vi "Process.vi"(8 "error in":errorcluster, 11 "Inst UI.RP100":refnum<class "Inst UI.RP100.lvclass">) -> (0 "error out":errorcluster, 3 "Inst UI.RP100 out":refnum<class "Inst UI.RP100.lvclass">)   [LabVIEW 2019, in "Inst UI.RP100.lvclass"]
doc: "---------------------------------------------------------------\nJKI State Machine Objects™\nhttp://jki.net/state-machine-objects/\nCopyright (C) 2005-2015, JKI <info@jki.net>\nALL RIGHTS RESERVEDJKI State Machine Objects (SMO) 1.0.0.5\nJKI - JKI\nCopyright (c) 2016, JKI"
uses:
  Inst UI.RP100.lvclass
  <vilib>/JKI/JKI SMO/SMO/SMO.lvclass
  <vilib>/JKI/JKI SMO/SMO.UI/SMO.UI.lvclass
  <userlib>/LevyLab/Instrument Framework/SMOs/Instrument/Instrument.lvclass
  Inst.RP100/Typedefs/Inst.RP100.getAll--Cluster.ctl
  Inst.RP100/Inst.RP100.lvclass
  <userlib>/LevyLab/Instrument Framework/SMOs/Instrument UI/Instrument UI.lvclass
  Inst UI.RP100.UI--Cluster.ctl
  <userlib>/LevyLab/Instrument Framework/SMOs/Configuration/Configuration.lvclass
  Inst.RP100/Typedefs/Inst.RP100.Configuration--Cluster.ctl
  <userlib>/LevyLab/Instrument Framework/SMOs/Instrument/Typedefs/Client Type--Enum.ctl
  <userlib>/LevyLab/Instrument Framework/SMOs/RemoteControl/Typedefs/Message--Cluster.ctl
  <userlib>/LevyLab/Instrument Framework/SMOs/RemoteControl/RemoteControl.lvclass
  09e9697b-516c-49fb-b2dc-692589121b6f.vi
  C:/Program Files (x86)/National Instruments/LabVIEW 2019/user.lib/LevyLab/Instrument Framework/SMOs/Instrument UI/Instrument UI.lvclass
  C:/Program Files (x86)/National Instruments/LabVIEW 2019/vi.lib/JKI/JKI SMO/SMO.UI/SMO.UI.lvclass
  C:/Program Files (x86)/National Instruments/LabVIEW 2019/vi.lib/JKI/JKI SMO/SMO/SMO.lvclass
  C:/Program Files (x86)/National Instruments/LabVIEW 2019/user.lib/LevyLab/Instrument Framework/Instrument Types/VSource/Instrument.VSource.lvclass
  C:/Program Files (x86)/National Instruments/LabVIEW 2019/user.lib/LevyLab/Instrument Framework/SMOs/Instrument/Instrument.lvclass
  Inst.RP100/Typedefs/Output State--Enum.ctl
  RP100/RP100.lvclass
  Inst.RP100/Typedefs/Output Channel--Enum.ctl
panel:
  in  "Go to Setpoint":bool
  in  "Enable Output":bool
  in  "Slew (V/s)":dbl=0.0001 min=0.0001 max=100.0 format="%#_6p"
  in  "Ch2 (V)":dbl min=-200.0 max=200.0
  in  "Ch1 (V)":dbl min=-200.0 max=200.0
  out "Bridge Titles":string="C\nC =\nLoss=\nV ="
  out "Bridge Status":string="Bridge:NaNpF\n0.000000nS\n0.000000V"
  out "Ch 2 status":string="Channel 2:Shorted\n0.0V\n0.0V\n0.0V\n0.0A"
  out "Ch 1 Status":string="Channel 1:Shorted\n0.0V\n0.0V\n0.0V\n0.0A"
  out "RP100 Titles":string="RP100\nState =\nLevel =\nSlew =\nMeasured V =\nMeasured I ="
  out "Status":string="SMO State: Stopped"
  out "version":string="vDevelopment"
  # "Razorbill Monitor & Control"
  # "Actions"
  # "Setpoints"
  # "RP100 Status"
  # "Bridge Status"
  # "SMO UI Template"
  # "For instructions on how to use the JKI State Machine Objects, examples and video tutorials, visit:\nhttp://jki.net/state-machine-objects/\n\nJKI State Machine Objects™\nhttp://jki.net/state-machine-objects/\nCopyright (C) 2005-2015, JKI <info@jki.net>\nALL RIGHTS RESERVED"
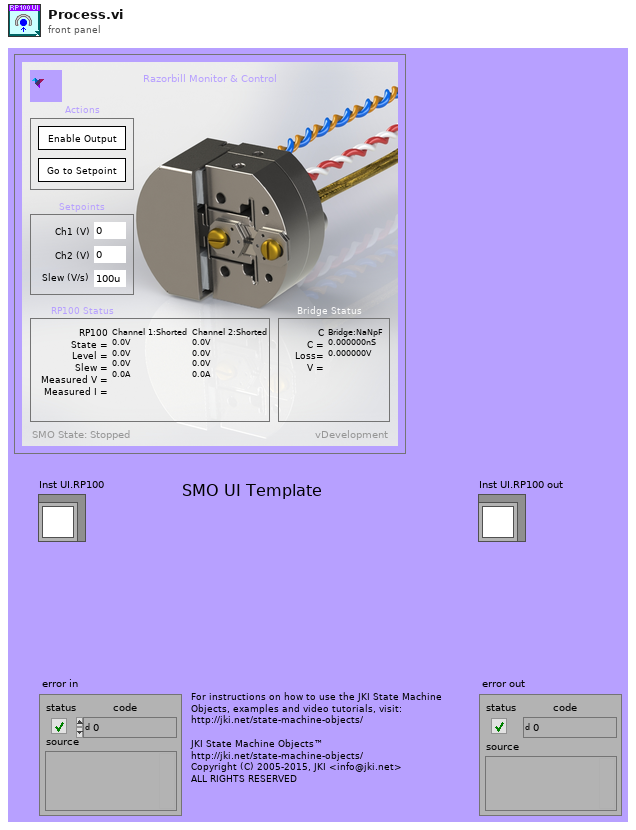
[diagram p1: front panel]
types:
  T1 = typedef "Inst.RP100.lvclass/Output State--Enum.ctl" = enum16{"Shorted", "Enabled"}
  T2 = typedef "Inst.RP100.lvclass/Output Channel--Enum.ctl" = enum16{"Output 1", "Output 2"}
  T3 = enum32{"invalid app kind", "Development System", "Run Time System", "Student Edition", "Embedded LabVIEW", "Evaluation", "Custom"}
  T4 = enum32{"Invalid", "Standard", "Closed", "Hidden", "Minimized", "Maximized"}
  T5 = typedef "Instrument.lvclass/Client Type--Enum.ctl" = enum16{"Remote", "Local"}
  T6 = typedef "RemoteControl.lvclass/Message--Cluster.ctl" = cluster{"Command":string, "Data":variant, "ID":string}
  T7 = typedef "Inst.RP100.lvclass/Inst.RP100.Configuration--Cluster.ctl" = cluster{"Example Setting 1":dbl, "Example Setting 2":dbl, "Example Setting 3":string}
  T8 = typedef "Inst.RP100.lvclass/Inst.RP100.getAll--Cluster.ctl" = cluster{"Output State Ch1":string, "Output State Ch2":string, "Level (V) Ch1":dbl, "Level (V) Ch2":dbl, "Slew (V/s) Ch1":dbl, "Slew (V/s) Ch2":dbl, "measured V (V) Ch1":dbl, "measured V (V) Ch2":dbl, "measured I (A) Ch1":dbl, "measured I (A) Ch2":dbl}
  T9 = typedef "Inst UI.RP100.lvclass/Inst UI.RP100.UI--Cluster.ctl" = cluster{"Ch1 (V)":dbl, "Ch2 (V)":dbl, "Slew (V/s)":dbl}
  T10 = cluster{"Core":cluster{"Current VI Reference":refnum<vi>, "Close Panel on Exit?":bool, "Last Error":cluster{"error":errorcluster, "previous state":string, "remaining states":string}, "Shutdown?":bool}, "Instrument UI":refnum<class "Inst UI.RP100.lvclass">, "Instrument":refnum<class "Inst.RP100.lvclass">, "Configuration":refnum<class "Configuration.lvclass">, "Config Cluster":T7, "getAll":T8, "UI Cluster":T9, "Message":T6}
  T11 = typedef "SMO.lvclass/SMOState --Enum.ctl" = enum16{"unknown", "Created", "Started", "Stopped"}
  T12 = cluster{"Current VI Reference":refnum<vi>, "Close Panel on Exit?":bool, "Last Error":cluster{"error":errorcluster, "previous state":string, "remaining states":string}, "Shutdown?":bool}
  T13 = typedef "SMO.lvclass/Protected Events.ctl" = cluster{"StopProcesses":refnum<user-event>, "AbortProcesses":refnum<user-event>, "Config Changed":refnum<user-event>, "Dependency":refnum<user-event>}
  T14 = typedef "Instrument.lvclass/PublicEvents--Cluster.ctl" = cluster{"MessageFromProcess":refnum<user-event>}
  T15 = typedef "Inst.RP100.lvclass/PublicEvents--Cluster.ctl" = cluster{"MessageFromProcess":refnum<user-event>}
  T16 = typedef "SMO.lvclass/Public Events.ctl" = cluster{"Error":refnum<user-event>, "State":refnum<user-event>, "Reserve State":refnum<user-event>}
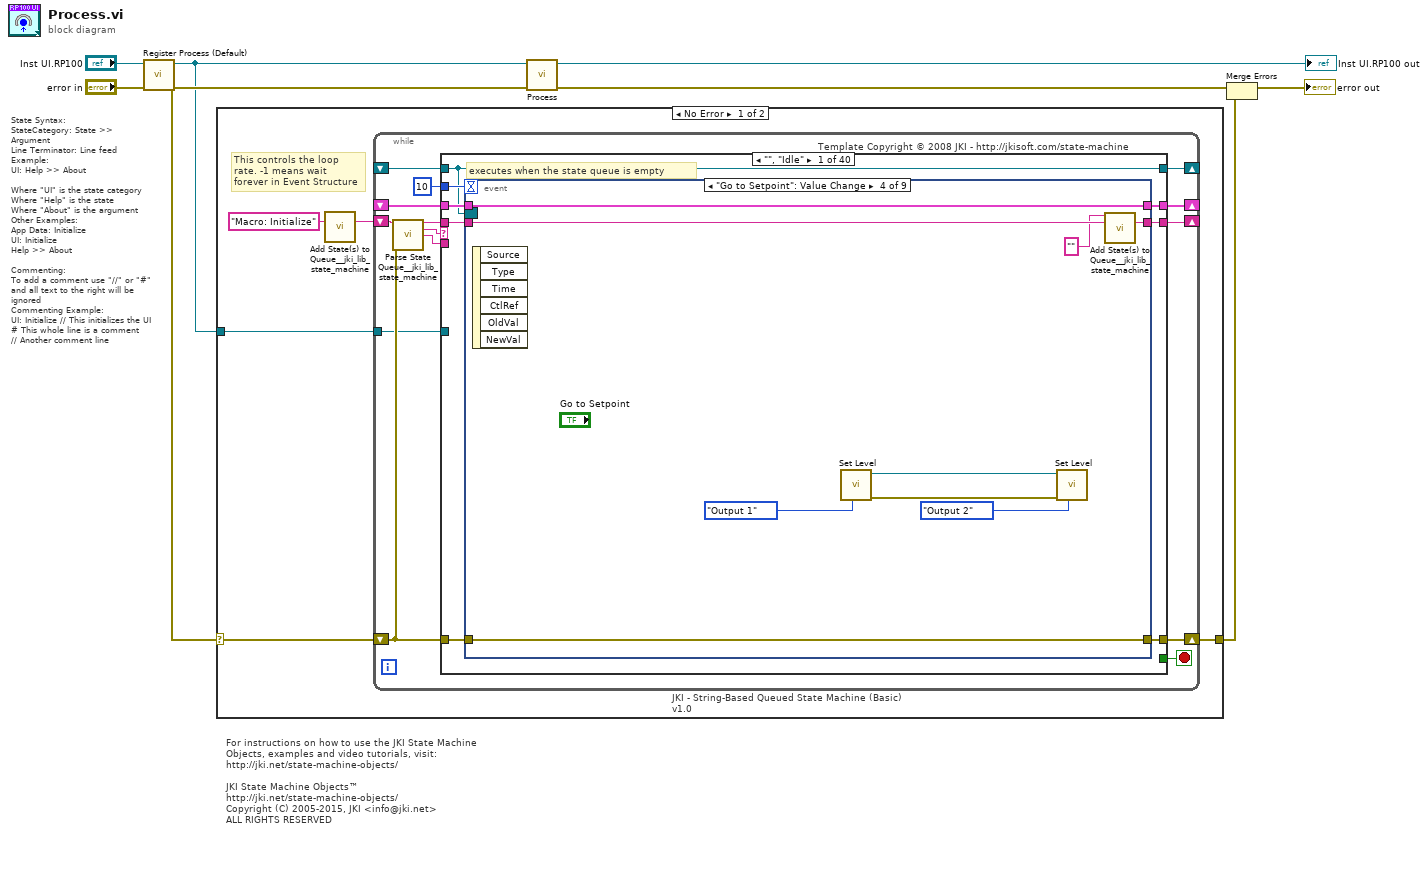
[diagram p0: block diagram]
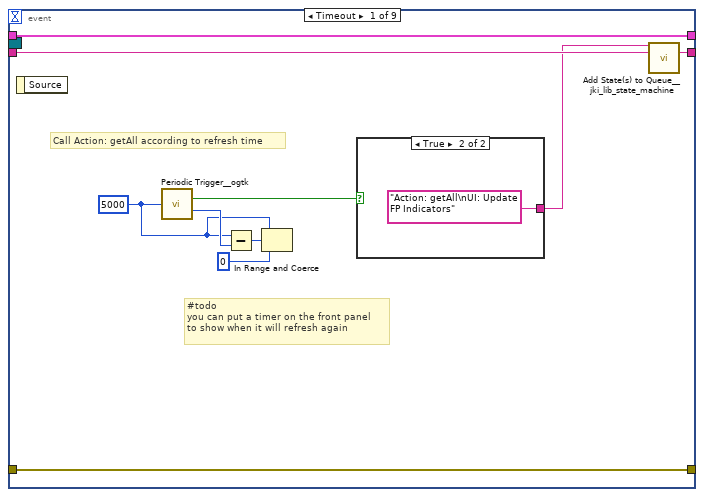
[diagram p2: hidden frame]
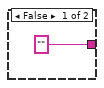
[diagram p3: hidden frame]
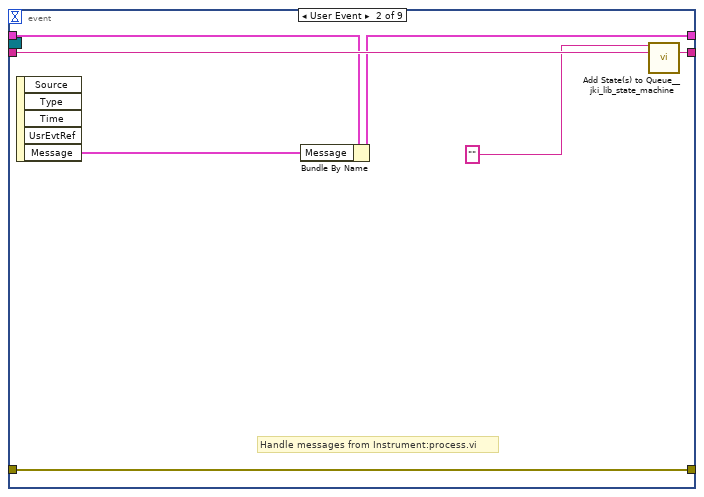
[diagram p4: hidden frame]
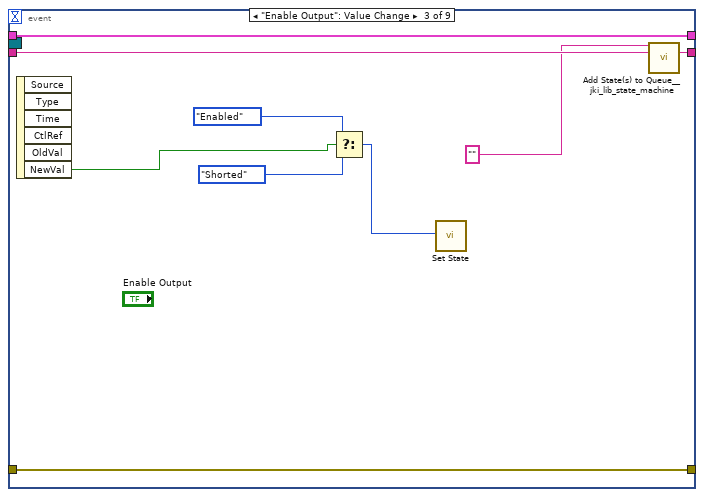
[diagram p5: hidden frame]
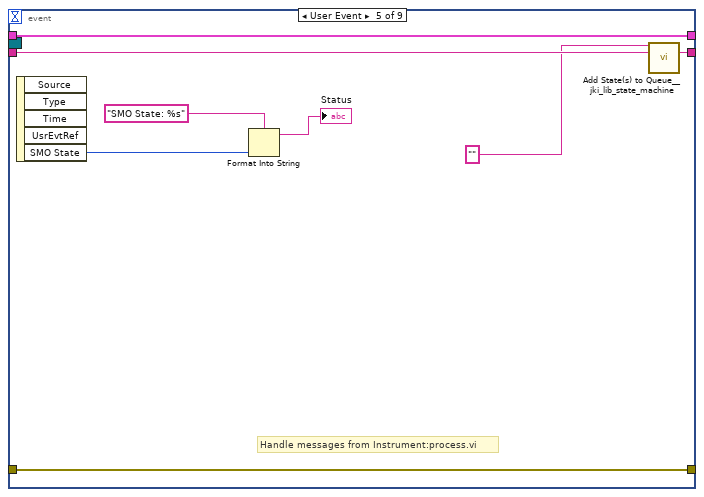
[diagram p6: hidden frame]
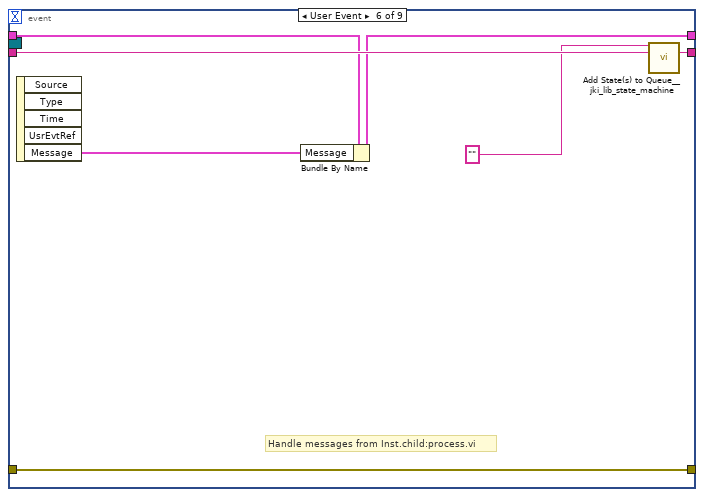
[diagram p7: hidden frame]
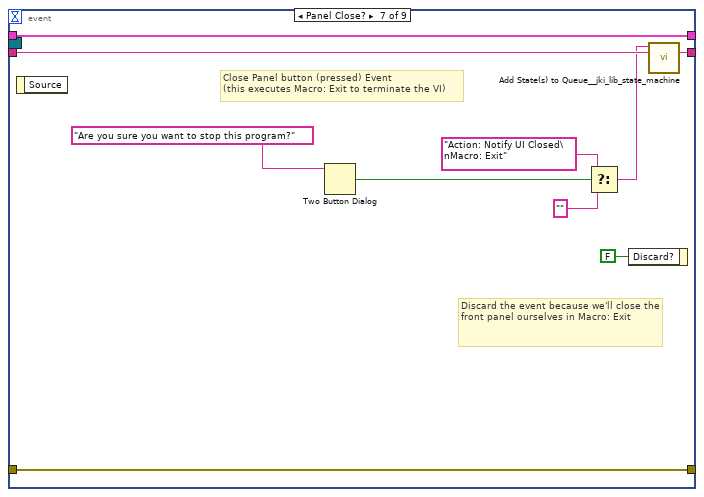
[diagram p8: hidden frame]
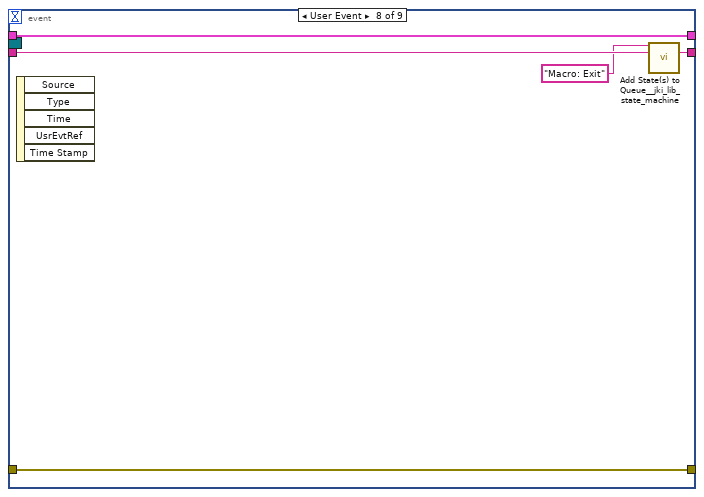
[diagram p9: hidden frame]
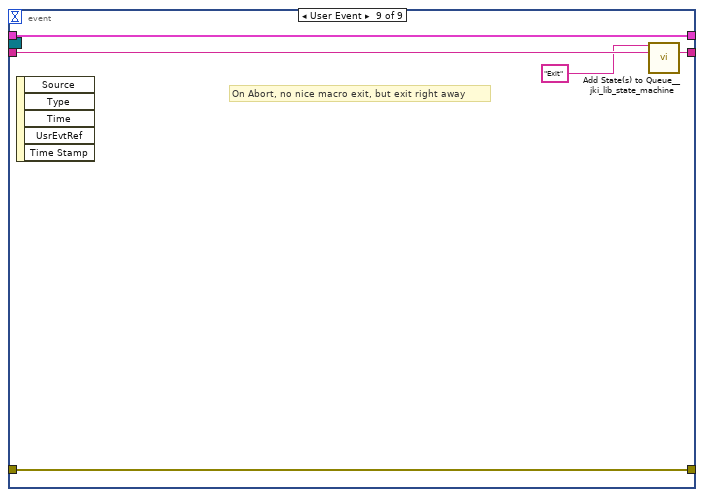
[diagram p10: hidden frame]
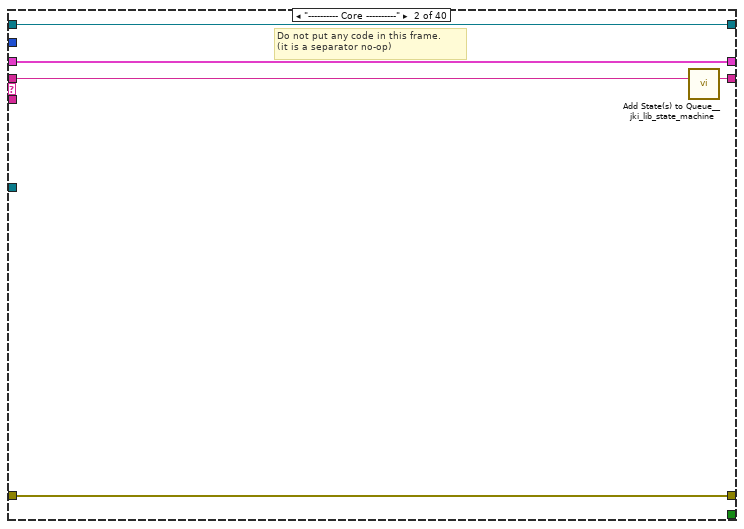
[diagram p11: hidden frame]
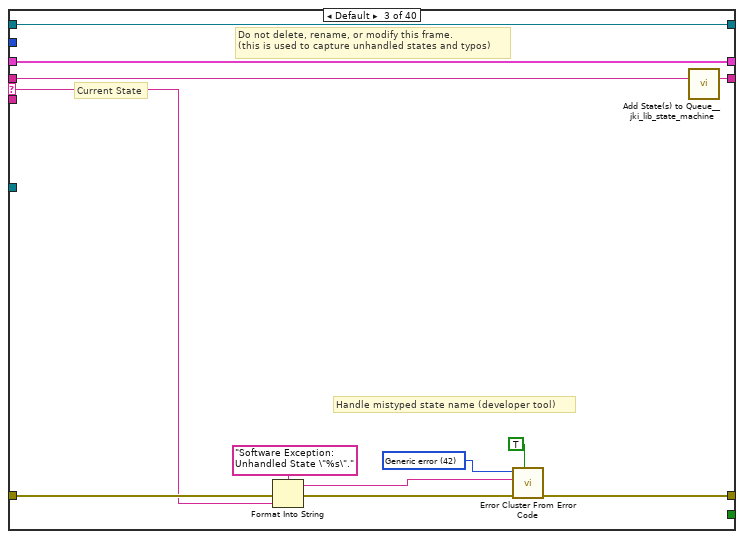
[diagram p12: hidden frame]
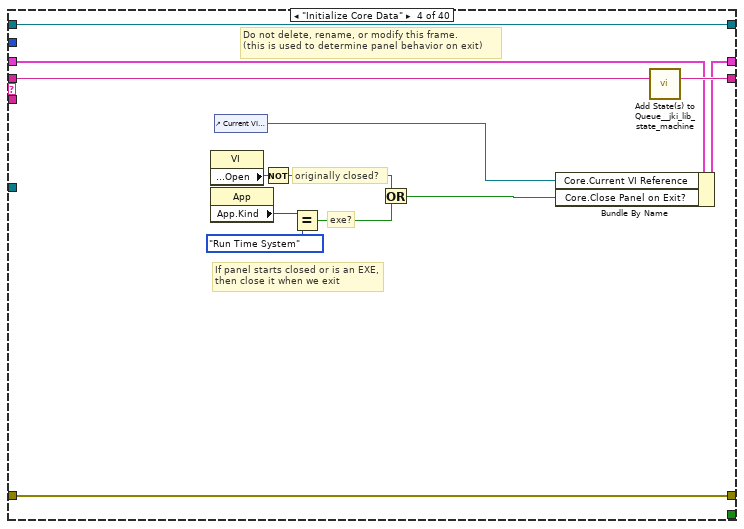
[diagram p13: hidden frame]
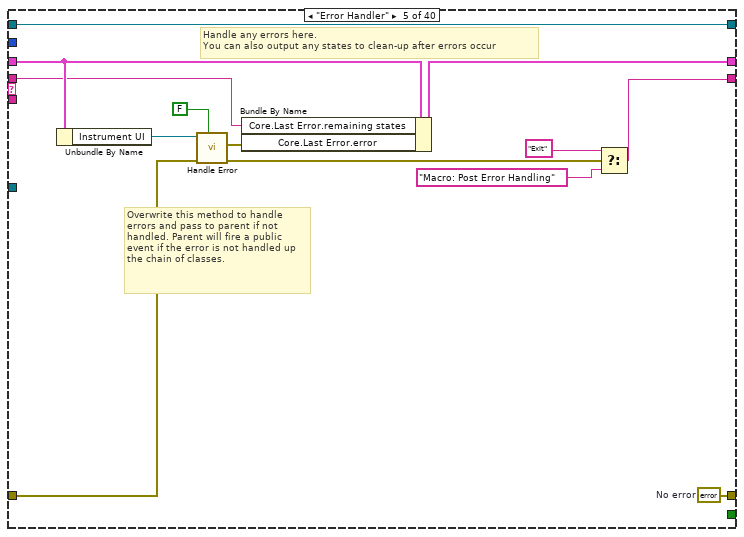
[diagram p14: hidden frame]
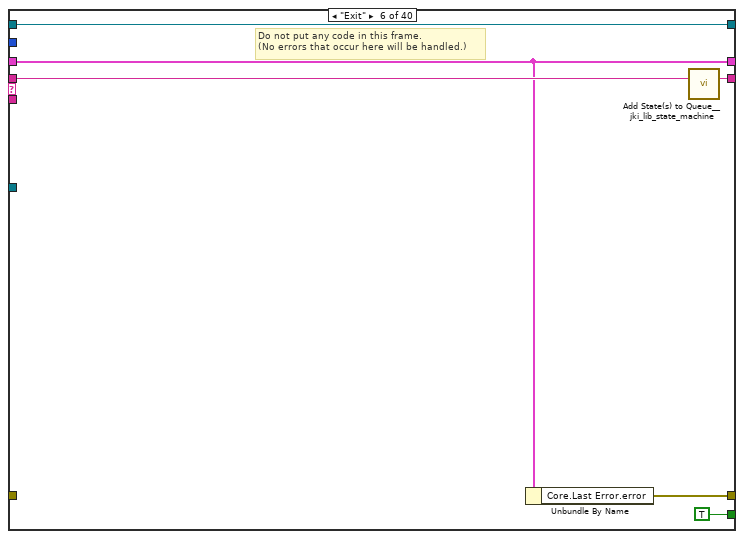
[diagram p15: hidden frame]
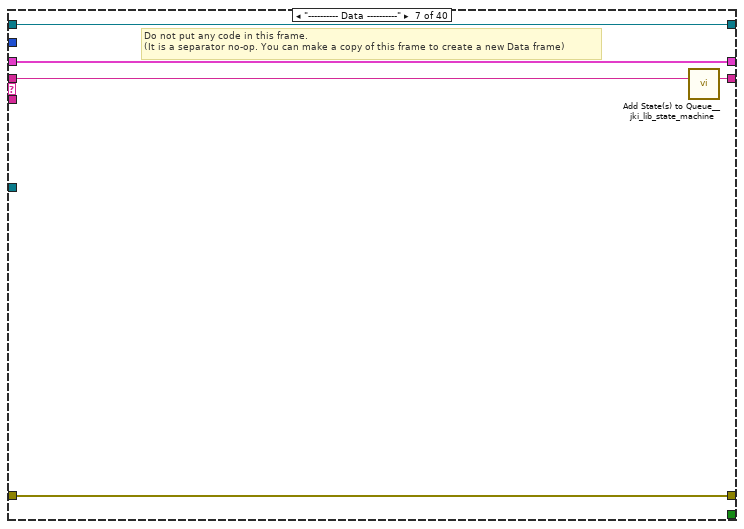
[diagram p16: hidden frame]
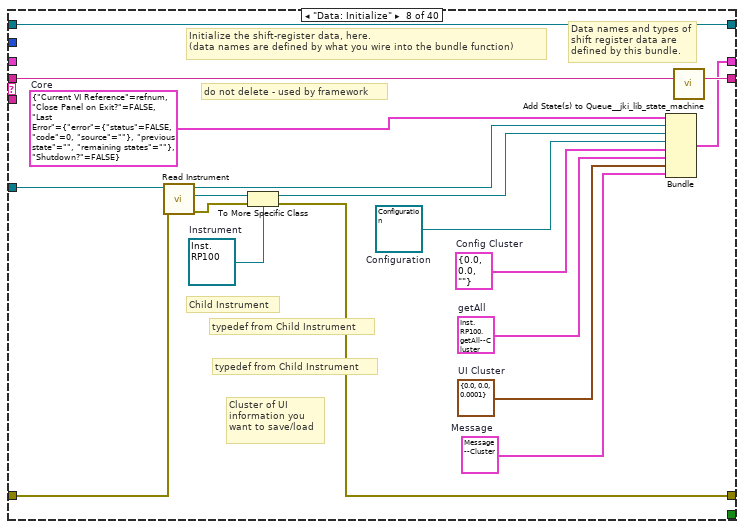
[diagram p17: hidden frame]
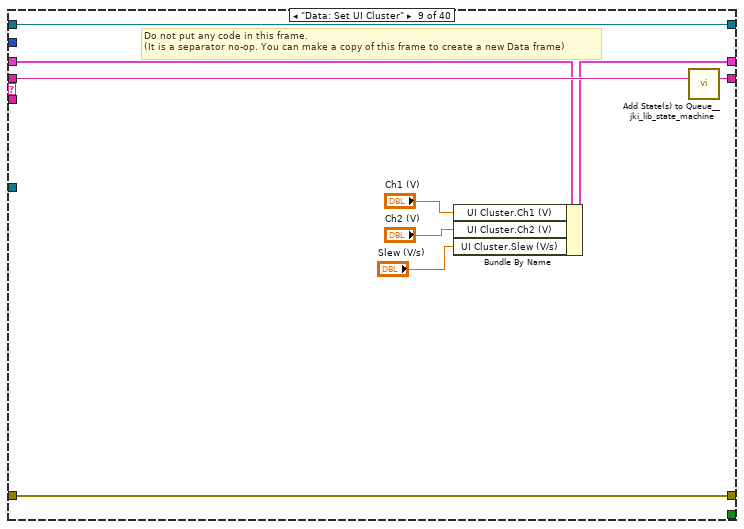
[diagram p18: hidden frame]
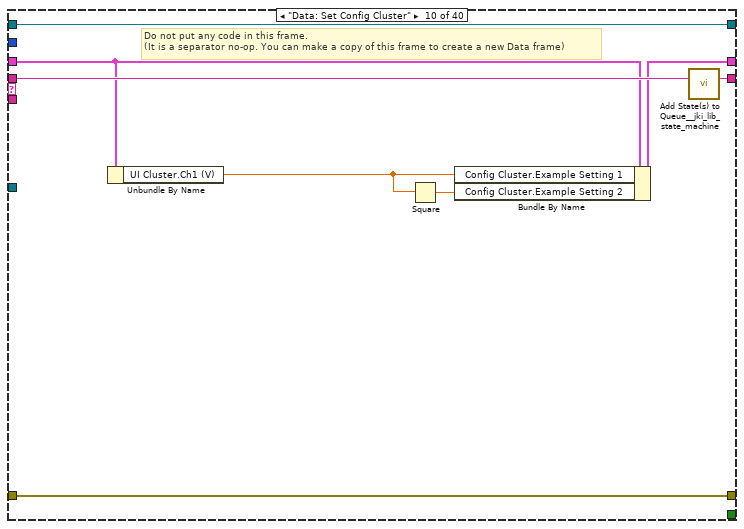
[diagram p19: hidden frame]
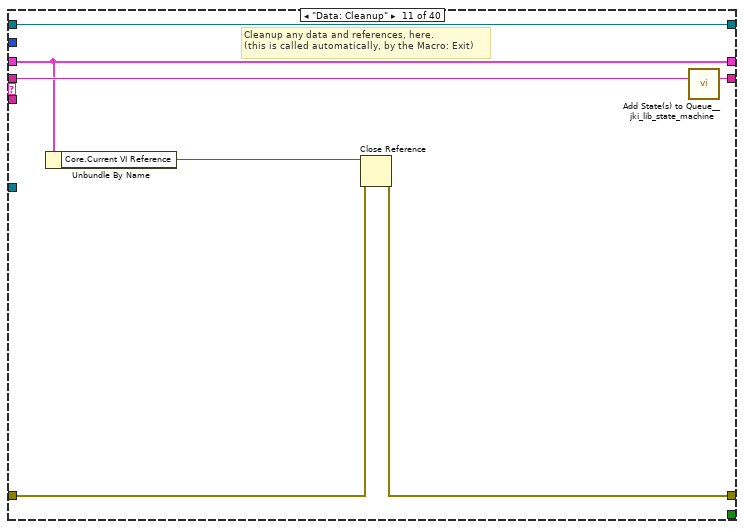
[diagram p20: hidden frame]
diagram:
  # "State Syntax:\nStateCategory: State >> Argument\nLine Terminator: Line feed\nExample:\nUI: Help >> About\n\nWhere \"UI\" is the state category\nWhere \"Help\" is the state\nWhere \"About\" is the argument\nOther Examples:\nApp Data: Initialize\nUI: Initialize\nHelp >> About\n\nCommenting:\nTo add a comment use \"//\" or \"#\" and all text to the right will be ignored\nCommenting Example:\nUI: Initialize // This initializes the UI\n# This whole line is a comment\n// Another comment line"
  # "For instructions on how to use the JKI State Machine Objects, examples and video tutorials, visit:\nhttp://jki.net/state-machine-objects/\n\nJKI State Machine Objects™\nhttp://jki.net/state-machine-objects/\nCopyright (C) 2005-2015, JKI <info@jki.net>\nALL RIGHTS RESERVED"
  n1 = call <vilib>:"Register Process (Default).vi"("error in (no error)"="error in", "SMO"="Inst UI.RP100") -> ("error out"=w5:errorcluster, "SelfRef"=w4:refnum<class "Inst UI.RP100.lvclass">)  [unwired: 8 in]
  n2 = case shown="No Error" w5 {
    selector: w5 -> [w10 w525]
    tunnel: w4 -> [w11 _]
    tunnel: [w9 w525] -> w1
    frame No Error {
      # "This controls the loop rate. -1 means wait forever in Event Structure"
      n3 = call <vilib>:"Add State(s) to Queue__jki_lib_state_machine.vi"("State(s) in (\"\")"="Macro: Initialize") -> ("States Out"=w13:string)  [unwired: 14 in]
      n4 = while "JKI - String-Based Queued State Machine (Basic) v1.0" {
        shift-right: [w20] -> _
        shift-left: _ -> [w19]
        shift-right: [w23] -> w9
        shift-left: w10 -> [w17]
        shift-right: [w22] -> _
        shift-left: w13 -> [w24]
        tunnel: w11 -> [w16]
        shift-right: [w15] -> _
        shift-left: _ -> [w14]
        stop <- w21 stop-if-true
        # "Template Copyright © 2008 JKI - http://jkisoft.com/state-machine"
        n5 = call <vilib>:"Parse State Queue__jki_lib_state_machine.vi"("State Queue"=w24, "Error In (no error)"=w17) -> ("Remaining States"=w26:string, "Current State"=w27:string, "Arguments"=w25:string)  [unwired: 11 in]
        n6 = case shown="\"\", \"Idle\"" w27 {
          selector: w27 -> [_ _ w114 _ _ _ _ _ _ _ _ _ _ _ _ _ _ _ _ _ _ _ _ _ _ _ _ _ _ _ _ _ _ _ _ _ _ _ _ _]
          tunnel: w26 -> [w35 w112 w118 w137 w141 w156 w161 w179 w188 w196 w203 w208 w220 w228 w255 w262 w278 w310 w319 w331 w341 w347 w362 w367 w378 w385 w390 w409 w415 w420 w435 w443 w455 w462 w469 w481 w494 w504 w514 w524]
          tunnel: w25 -> [_ _ _ _ _ _ _ _ _ _ _ _ _ _ _ w256 w272 _ _ _ _ _ _ _ _ _ _ _ _ _ _ _ _ _ _ _ _ _ _ _]
          tunnel: w19 -> [w33 w109 w116 w128 w144 w152 w158 _ w184 w192 w197 w205 w218 w224 w251 w260 w274 w307 w315 w321 w338 w344 w349 w364 w375 w380 w387 w407 w413 w417 w428 w440 w446 w457 w463 w473 w488 w496 w509 w519]
          tunnel: [w32 w110 w120 w134 w146 w151 w159 w166 w186 w194 w199 w206 w215 w226 w252 w257 w275 w308 w317 w329 w339 w345 w360 w365 w369 w381 w388 w404 w410 w418 w421 w438 w447 w459 w464 w478 w491 w501 w505 w515] -> w23
          tunnel: w17 -> [w31 w110 w119 w134 w140 _ w159 w163 w186 w194 w200 w206 w216 w226 w252 w258 w276 w308 w317 w329 w339 w345 w360 w365 w370 w382 w388 w394 w411 w418 w430 w436 w448 w459 w465 w474 w483 w497 w506 w516]
          tunnel: [w34 w111 w117 w136 w138 w155 w160 w178 w187 w195 w202 w207 w219 w227 w254 w261 w277 w309 w318 w330 w340 w346 w361 w366 w377 w384 w389 w408 w414 w419 w434 w442 w454 w461 w468 w480 w493 w503 w513 w523] -> w22
          tunnel: [_ _ _ _ _ TRUE _ _ _ _ _ _ _ _ _ _ _ _ _ _ _ _ _ _ _ _ _ _ _ _ _ _ _ _ _ _ _ _ _ _] -> w21
          tunnel: [w30 w109 w116 w135 w143 w152 w158 w177 w183 w191 w197 w205 w218 w224 w251 w260 w274 w307 w315 w322 w338 w344 w349 w364 w375 w380 w387 w407 w413 w417 w432 w440 w444 w456 w463 w475 w489 w498 w510 w520] -> w20
          tunnel: 10 ("Timeout") -> [w29 _ _ _ _ _ _ _ _ _ _ _ _ _ _ _ _ _ _ _ _ _ _ _ _ _ _ _ _ _ _ _ _ _ _ _ _ _ _ _]
          tunnel: w16 -> [_ _ _ _ _ _ _ w164 _ _ _ _ _ _ _ _ _ _ _ _ _ _ _ _ _ _ _ _ _ _ _ _ _ _ _ _ _ _ _ _]
          tunnel: [w28 w108 w113 w125 w150 w153 w157 w176 w185 w193 w198 w204 w217 w225 w253 w259 w271 w306 w316 w328 w337 w343 w354 w363 w376 w383 w386 w406 w412 w416 w433 w441 w453 w460 w467 w479 w492 w502 w512 w522] -> w15
          tunnel: w14 -> [w28 w108 w113 w125 w150 w153 w157 w176 w185 w193 w198 w204 w217 w225 w253 w259 w271 w306 w316 w328 w337 w343 w354 w363 w376 w383 w386 _ w412 w416 w433 w441 w453 w460 w467 w479 w492 w502 w512 w522]
          frame "", "Idle" {
            # "executes when the state queue is empty"
            n7 = event shown="[3] \"Go to Setpoint\": Value Change" {
              selector: w28 -> [_ _ _ _ _ _ _ _ _]
              dyn-events: _ -> [_ _ _ _ _ _ _ _ _]
              timeout: w29 -> [_ _ _ _ _ _ _ _ _]
              tunnel: w35 -> [w45 w54 w63 w72 w80 w87 w97 w102 w107]
              tunnel: [w44 w53 w62 w71 w79 w86 w96 w101 w106] -> w34
              tunnel: w33 -> [w42 w51 w59 w69 w76 w84 w94 w99 w104]
              tunnel: [w43 w52 w61 w70 w78 w85 w93 w100 w105] -> w32
              tunnel: w31 -> [w43 w52 w61 w70 w78 w85 w93 w100 w105]
              tunnel: [w42 w50 w59 w69 w76 w83 w94 w99 w104] -> w30
              event Timeout {
                w37 = u32 5000 ("time (ms)")
                # "#todo\nyou can put a timer on the front panel\nto show when it will refresh again"
                # "Call Action: getAll according to refresh time"
                n8 = event-data() -> ()  [unwired: 1 in, 1 out]
                n9 = call <userlib>:"Periodic Trigger__ogtk.vi"("time (ms)"=w37) -> ("Triggered"=w40:bool, "timer value"=w39:u32)  [unwired: 12 in, 1 out]
                n10 = Subtract(x=w37, y=w39) -> (x-y=w38:u32)
                n11 = In Range and Coerce(upper limit=w37, x=w38, lower limit=u32 0) -> ()  [unwired: 2 out]
                n12 = case shown="True" w40 {
                  tunnel: ["" ("State(s) in Front (\"\")") "Action: getAll\nUI: Update FP Indicators" ("State(s) in Front (\"\")")] -> w41
                  frame False {
                  }
                  frame True {
                  }
                }
                n13 = call <vilib>:"Add State(s) to Queue__jki_lib_state_machine.vi"("State(s) in Front (\"\")"=w41, "State(s) in (\"\")"=w45) -> ("States Out"=w44:string)  [unwired: 13 in]
              }
              event User Event {
                # "Handle messages from Instrument:process.vi"
                n14 = event-data() -> ("Message"=w48:T6)  [unwired: 1 in, 4 out]
                n15 = Bundle By Name(cluster=w51, "Message"=w48) -> (w50:T10)
                n16 = call <vilib>:"Add State(s) to Queue__jki_lib_state_machine.vi"("State(s) in Front (\"\")"="" ("State(s) in Front (\"\")"), "State(s) in (\"\")"=w54) -> ("States Out"=w53:string)  [unwired: 13 in]
              }
              event "Enable Output": Value Change {
                n17 = event-data() -> ("NewVal"=w55:bool)  [unwired: 1 in, 5 out]
                n18 = Select(t=Output_State--Enum."Enabled" ("Output"), s=w55, f=Output_State--Enum."Shorted" ("Output")) -> (s? t:f=w56:T1)
                n19 = call-dynamic "Set State.vi"("Output"=w56) -> ()  [unwired: 9 in, 2 out]
                n20 = call <vilib>:"Add State(s) to Queue__jki_lib_state_machine.vi"("State(s) in Front (\"\")"="" ("State(s) in Front (\"\")"), "State(s) in (\"\")"=w63) -> ("States Out"=w62:string)  [unwired: 13 in]
              }
              event "Go to Setpoint": Value Change {
                n21 = event-data() -> ()  [unwired: 1 in, 6 out]
                n22 = call-dynamic "Set Level.vi"("Output Channel"=Output_Channel--Enum."Output 1") -> ("error out"=w64:errorcluster, "RP100 out"=w67:refnum<class "RP100.lvclass">)  [unwired: 9 in]
                n23 = call-dynamic "Set Level.vi"("Output Channel"=Output_Channel--Enum."Output 2", "error in (no error)"=w64, "RP100 in"=w67) -> ()  [unwired: 7 in, 2 out]
                n24 = call <vilib>:"Add State(s) to Queue__jki_lib_state_machine.vi"("State(s) in Front (\"\")"="" ("State(s) in Front (\"\")"), "State(s) in (\"\")"=w72) -> ("States Out"=w71:string)  [unwired: 13 in]
              }
              event User Event {
                # "Handle messages from Instrument:process.vi"
                n25 = event-data() -> ("SMO State"=w74:T11)  [unwired: 1 in, 4 out]
                n26 = Format Into String(format string="SMO State: %s", w74) -> (resulting string=→"Status":string)  [unwired: 2 in, 1 out]
                n27 = call <vilib>:"Add State(s) to Queue__jki_lib_state_machine.vi"("State(s) in Front (\"\")"="" ("State(s) in Front (\"\")"), "State(s) in (\"\")"=w80) -> ("States Out"=w79:string)  [unwired: 13 in]
              }
              event User Event {
                # "Handle messages from Inst.child:process.vi"
                n28 = event-data() -> ("Message"=w81:T6)  [unwired: 1 in, 4 out]
                n29 = Bundle By Name(cluster=w84, "Message"=w81) -> (w83:T10)
                n30 = call <vilib>:"Add State(s) to Queue__jki_lib_state_machine.vi"("State(s) in Front (\"\")"="" ("State(s) in Front (\"\")"), "State(s) in (\"\")"=w87) -> ("States Out"=w86:string)  [unwired: 13 in]
              }
              event Panel Close? {
                # "Discard the event because we'll close the front panel ourselves in Macro: Exit"
                # "Close Panel button (pressed) Event\n(this executes Macro: Exit to terminate the VI)"
                n31 = event-data() -> ()  [unwired: 1 in, 1 out]
                n32 = Two Button Dialog(message="Are you sure you want to stop this program?") -> (T button?=w92:bool)  [unwired: 2 in]
                n33 = Select(t="Action: Notify UI Closed\nMacro: Exit", s=w92, f="") -> (s? t:f=w89:string)
                n34 = event-data("Discard?"=FALSE) -> ()  [unwired: 1 in, 1 out]
                n35 = call <vilib>:"Add State(s) to Queue__jki_lib_state_machine.vi"("State(s) in Front (\"\")"=w89, "State(s) in (\"\")"=w97) -> ("States Out"=w96:string)  [unwired: 13 in]
              }
              event User Event {
                n36 = event-data() -> ()  [unwired: 1 in, 5 out]
                n37 = call <vilib>:"Add State(s) to Queue__jki_lib_state_machine.vi"("State(s) in Front (\"\")"="Macro: Exit", "State(s) in (\"\")"=w102) -> ("States Out"=w101:string)  [unwired: 13 in]
              }
              event User Event {
                # "On Abort, no nice macro exit, but exit right away"
                n38 = event-data() -> ()  [unwired: 1 in, 5 out]
                n39 = call <vilib>:"Add State(s) to Queue__jki_lib_state_machine.vi"("State(s) in Front (\"\")"="Exit", "State(s) in (\"\")"=w107) -> ("States Out"=w106:string)  [unwired: 13 in]
              }
            }
          }
          frame "---------- Core ----------" {
            # "Do not put any code in this frame.\n(it is a separator no-op)"
            n40 = call <vilib>:"Add State(s) to Queue__jki_lib_state_machine.vi"("State(s) in (\"\")"=w112) -> ("States Out"=w111:string)  [unwired: 14 in]
          }
          frame Default {
            w123 = 42 items=["No error", "Argument error", "Memory is full", "Out of zone", "End of file", "File already open", "Generic file I/O error", "File not found", "File permission error", "Disk is full", "Duplicate path", "Too many files open", "System feature not enabled", "Resource file not found", "Cannot add resource", "Resource not found", "Image not found", "Image memory error", "Pen does not exist", "Config type invalid", "Config token not found", "Config parse error", "Config memory error", "Bad external code format", "Bad external code offset", "External code not present", "Null window", "Destroy window error", "Null menu", "Print aborted", "Bad print record", "Print driver error", "Windows error during printing", "Memory error during printing", "Print dialog error", "Generic print error", "Invalid device refnum", "Device not found", "Device parameter error", "Device unit error", "Cannot open device", "Device call aborted", "Generic error", "Cancelled by user", "Object ID too low", "Object ID too high", "Object not in heap", "Unknown heap", "Unknown object (invalid DefProc)", "Unknown object (DefProc not in table)", "Message out of range", "Invalid (null) method", "Unknown message", "Manager call not supported", "Bad address", "Network operation in progress", "Network operation timed out", "Connection is busy", "Network attribute not supported", "Network error", "Address in use", "System out of memory", "Connection aborted", "Connection refused", "Not connected", "Already connected", "Connection closed", "Initialization error (interapplication manager)", "Bad occurrence", "Wait on unbound occurrence handler", "Occurrence queue overflow", "Datalog type conflict", "Unused", "Unrecognized type (interapplication manager)", "Memory corrupt", "Failed to make temporary DLL", "Old CIN version", "Drag socket not found", "Failed to load drop-object", "Failed to register OLE object", "Failed to release OLE object", "Format specifier type mismatch", "Unknown format specifier", "Too few format specifiers", "Too many format specifiers", "Scan failed", "Newer CIN version", "Error converting to variant", "Runtime menu error", "Password tampered", "Variant attribute not found", "Incompatible variant data type", "Event data is not available", "Event Store is not present", "Occurrence is not found", "Event Queue is not created", "Event info is not available", "Refnum passed is NULL", "Error retrieving Class GUID", "Error retrieving CoClass GUID", "Error retrieving TypeLib GUID.", "Bad built application magic bytes.", "Specific driver is different from the specific driver associated with the Logical Name.", "There is no session opened to the class driver.", "Max Error", "MAX - Error with config objects", "MAX - Error loading configuration", "MAX - Group not supported"]
            # "Current State"
            # "Do not delete, rename, or modify this frame.\n(this is used to capture unhandled states and typos)"
            # "Handle mistyped state name (developer tool)"
            n41 = Format Into String(format string="Software Exception: Unhandled State \"%s\"." ("message"), error in=w119, w114) -> (resulting string=w122:string, error out=w121:errorcluster)  [unwired: 1 in]
            n42 = call <vilib>:"Error Cluster From Error Code.vi"("show call chain? (False)"=TRUE, "error in (no error)"=w121, "error message (\"\")"=w122, "error code (0)"=w123) -> ("error out"=w120:errorcluster)  [unwired: 5 in]
            n43 = call <vilib>:"Add State(s) to Queue__jki_lib_state_machine.vi"("State(s) in (\"\")"=w118) -> ("States Out"=w117:string)  [unwired: 14 in]
          }
          frame "Initialize Core Data" {
            # "Do not delete, rename, or modify this frame.\n(this is used to determine panel behavior on exit)"
            # "originally closed?"
            # "exe?"
            # "If panel starts closed or is an EXE, then close it when we exit"
            n44 = property class="VI"() -> ("Front Panel.Open"=w133:bool)  [unwired: 2 in, 2 out]
            n45 = property class="App"() -> ("App.Kind"=w132:T3)  [unwired: 2 in, 2 out]
            n46 = control-ref of="Current VI Reference"() -> (w126:refnum<vi>)
            n47 = Not(x=w133) -> (.not. x?=w130:bool)
            n48 = Equal?(x=w132, y=T3."Run Time System" ("Application:Kind")) -> (x = y?=w129:bool)
            n49 = Or(x=w130, y=w129) -> (x .or. y?=w127:bool)
            n50 = Bundle By Name(cluster=w128, "Core.Current VI Reference"=w126, "Core.Close Panel on Exit?"=w127) -> (w135:T10)
            n51 = call <vilib>:"Add State(s) to Queue__jki_lib_state_machine.vi"("State(s) in (\"\")"=w137) -> ("States Out"=w136:string)  [unwired: 14 in]
          }
          frame "Error Handler" {
            w146 = errorcluster {"status"=FALSE, "code"=0, "source"=""}  # No error
            # "Overwrite this method to handle errors and pass to parent if not handled. Parent will fire a public event if the error is not handled up the chain of classes."
            # "Handle any errors here.\nYou can also output any states to clean-up after errors occur"
            n52 = Unbundle By Name(w144) -> ("Instrument UI"=w149:refnum<class "Inst UI.RP100.lvclass">)
            n53 = call-dynamic "Handle Error.vi"("Stop on Unhandled Error (T)"=FALSE, "error in"=w140, "SMO"=w149) -> ("handling error"=w147:errorcluster, "Unhandled error"=w145:errorcluster)  [unwired: 6 in, 1 out]
            n54 = Bundle By Name(cluster=w144, "Core.Last Error.remaining states"=w141, "Core.Last Error.error"=w145) -> (w143:T10)
            n55 = Select(t="Exit", s=w147, f="Macro: Post Error Handling") -> (s? t:f=w138:string)
          }
          frame "Exit" {
            # "Do not put any code in this frame.\n(No errors that occur here will be handled.)"
            n56 = Unbundle By Name(w152) -> ("Core.Last Error.error"=w151:errorcluster)
            n57 = call <vilib>:"Add State(s) to Queue__jki_lib_state_machine.vi"("State(s) in (\"\")"=w156) -> ("States Out"=w155:string)  [unwired: 14 in]
          }
          frame "---------- Data ----------" {
            # "Do not put any code in this frame.\n(It is a separator no-op. You can make a copy of this frame to create a new Data frame)"
            n58 = call <vilib>:"Add State(s) to Queue__jki_lib_state_machine.vi"("State(s) in (\"\")"=w161) -> ("States Out"=w160:string)  [unwired: 14 in]
          }
          frame "Data: Initialize" {
            w162 = T6 {"Command"="", "Data"=variant, "ID"=""}  # Message
            w165 = refnum<class "Configuration.lvclass"> refnum  # Configuration
            w168 = T7 {"Example Setting 1"=0.0, "Example Setting 2"=0.0, "Example Setting 3"=""}  # Config Cluster
            w170 = T9 {"Ch1 (V)"=0.0, "Ch2 (V)"=0.0, "Slew (V/s)"=0.0001}  # UI Cluster
            w172 = refnum<class "Inst.RP100.lvclass"> refnum  # Instrument
            w174 = T8 {"Output State Ch1"="", "Output State Ch2"="", "Level (V) Ch1"=0.0, "Level (V) Ch2"=0.0, "Slew (V/s) Ch1"=0.0, "Slew (V/s) Ch2"=0.0, "measured V (V) Ch1"=0.0, "measured V (V) Ch2"=0.0, "measured I (A) Ch1"=0.0, "measured I (A) Ch2"=0.0}  # getAll
            w175 = T12 {"Current VI Reference"=refnum, "Close Panel on Exit?"=FALSE, "Last Error"={"error"={"status"=FALSE, "code"=0, "source"=""}, "previous state"="", "remaining states"=""}, "Shutdown?"=FALSE}  # Core
            # "typedef from Child Instrument"
            # "Cluster of UI\ninformation you\nwant to save/load"
            # "Child Instrument"
            # "typedef from Child Instrument"
            # "do not delete - used by framework"
            # "Data names and types of shift register data are defined by this bundle."
            # "Initialize the shift-register data, here.\n(data names are defined by what you wire into the bundle function)"
            n59 = call <userlib>:"Read Instrument.vi"("error in (no error)"=w163, "Instrument UI in"=w164) -> ("error out"=w169:errorcluster, "Instrument"=w171:refnum<class "Instrument.lvclass">, "Instrument UI"=w173:refnum<class "Inst UI.RP100.lvclass">)  [unwired: 7 in]
            n60 = To More Specific Class(target class=w172, reference=w171, error in=w169) -> (specific class reference=w167:refnum<class "Inst.RP100.lvclass">, error out=w166:errorcluster)
            n61 = Bundle("Core"=w175, "Instrument UI"=w173, "Instrument"=w167, "Configuration"=w165, "Config Cluster"=w168, "getAll"=w174, "UI Cluster"=w170, "Message"=w162) -> (w177:T10)  [unwired: 1 in]
            n62 = call <vilib>:"Add State(s) to Queue__jki_lib_state_machine.vi"("State(s) in (\"\")"=w179) -> ("States Out"=w178:string)  [unwired: 14 in]
          }
          frame "Data: Set UI Cluster" {
            # "Do not put any code in this frame.\n(It is a separator no-op. You can make a copy of this frame to create a new Data frame)"
            n63 = Bundle By Name(cluster=w184, "UI Cluster.Ch1 (V)"="Ch1 (V)", "UI Cluster.Ch2 (V)"="Ch2 (V)", "UI Cluster.Slew (V/s)"="Slew (V/s)") -> (w183:T10)
            n64 = call <vilib>:"Add State(s) to Queue__jki_lib_state_machine.vi"("State(s) in (\"\")"=w188) -> ("States Out"=w187:string)  [unwired: 14 in]
          }
          frame "Data: Set Config Cluster" {
            # "Do not put any code in this frame.\n(It is a separator no-op. You can make a copy of this frame to create a new Data frame)"
            n65 = Unbundle By Name(w192) -> ("UI Cluster.Ch1 (V)"=w190:dbl)
            n66 = Square(x=w190) -> (x^2=w189:dbl)
            n67 = Bundle By Name(cluster=w192, "Config Cluster.Example Setting 1"=w190, "Config Cluster.Example Setting 2"=w189) -> (w191:T10)
            n68 = call <vilib>:"Add State(s) to Queue__jki_lib_state_machine.vi"("State(s) in (\"\")"=w196) -> ("States Out"=w195:string)  [unwired: 14 in]
          }
          frame "Data: Cleanup" {
            # "Cleanup any data and references, here.\n(this is called automatically, by the Macro: Exit)"
            n69 = Unbundle By Name(w197) -> ("Core.Current VI Reference"=w201:refnum<vi>)
            n70 = Close Reference(reference=w201, error in (no error)=w200) -> (error out=w199:errorcluster)
            n71 = call <vilib>:"Add State(s) to Queue__jki_lib_state_machine.vi"("State(s) in (\"\")"=w203) -> ("States Out"=w202:string)  [unwired: 14 in]
          }
          frame "---------- UI ----------" {
            # "Do not put any code in this frame.\n(It is a separator no-op. You can make a copy of this frame to create a new UI frame)"
            n72 = call <vilib>:"Add State(s) to Queue__jki_lib_state_machine.vi"("State(s) in (\"\")"=w208) -> ("States Out"=w207:string)  [unwired: 14 in]
          }
          frame "UI: Initialize" {
            # "size window to decoration box on front panel"
            # "Initialize the User Interface, here.\n(this is called automatically, by the Macro: Init)"
            n73 = call <userlib>:"MGI Get Executable Version.vi"() -> ("Version"=w213:string)  [unwired: 7 in]
            n74 = Format Into String(format string="v%s", w213) -> (resulting string=→"version":string)  [unwired: 2 in, 1 out]
            n75 = call <userlib>:"Fit VI window to Largest Dec__ogtk.vi"("error in (no error)"=w216, "border spacing (2 px)"=0) -> ("error out"=w215:errorcluster)  [unwired: 4 in, 1 out]
            n76 = call <vilib>:"Add State(s) to Queue__jki_lib_state_machine.vi"("State(s) in (\"\")"=w220) -> ("States Out"=w219:string)  [unwired: 14 in]
            "Bridge Titles" <- "\nC =\nLoss =\nV =" ("Status 7")
            "RP100 Titles" <- "\nState =\nLevel =\nSlew =\nMeasured V =\nMeasured I =" ("Status 2")
          }
          frame "UI: Update FP Controls" {
            # "Do not put any code in this frame.\n(It is a separator no-op. You can make a copy of this frame to create a new UI frame)"
            n77 = Unbundle By Name(w224) -> ("UI Cluster.Ch1 (V)"=w223:dbl, "UI Cluster.Ch2 (V)"=w222:dbl, "UI Cluster.Slew (V/s)"=w221:dbl)
            n78 = local write "Ch1 (V)"(w223) -> ()
            n79 = local write "Ch2 (V)"(w222) -> ()
            n80 = local write "Slew (V/s)"(w221) -> ()
            n81 = call <vilib>:"Add State(s) to Queue__jki_lib_state_machine.vi"("State(s) in (\"\")"=w228) -> ("States Out"=w227:string)  [unwired: 14 in]
          }
          frame "UI: Update FP Indicators" {
            n82 = Unbundle By Name(w251) -> ("getAll"=w232:T8)
            n83 = Unbundle By Name(w232) -> ("Output State Ch1"=w250:string, "Level (V) Ch1"=w249:dbl, "Slew (V/s) Ch1"=w248:dbl, "measured V (V) Ch1"=w247:dbl, "measured I (A) Ch1"=w246:dbl, "Output State Ch2"=w245:string, "Level (V) Ch2"=w244:dbl, "Slew (V/s) Ch2"=w243:dbl, "measured V (V) Ch2"=w242:dbl, "measured I (A) Ch2"=w241:dbl, "bridge C (pF)"=w240, "bridge Loss (nS)"=w239, "bridge exc (V)"=w238)
            n84 = Format Into String(format string="%s\\n%.1pV\\n%.1pV\\n%.1pV\\n%.1pA", initial string="Channel 1:\n" ("Ch 1 Status"), w250, w249, w248, w247, w246) -> (resulting string=→"Ch 1 Status":string)  [unwired: 1 in, 1 out]
            n85 = Format Into String(initial string="Channel 2:\n" ("Ch 2 status"), w245, w244, w243, w242, w241) -> (resulting string=→"Ch 2 status":string)  [unwired: 2 in, 1 out]
            n86 = Format Into String(format string="%.1fpF\\n%.1fnS\\n%.1pV" ("Status 6"), initial string="\n" ("Ch 2 status"), w240, w239, w238) -> (resulting string=→"Bridge Status":string)  [unwired: 1 in, 1 out]
            n87 = call <vilib>:"Add State(s) to Queue__jki_lib_state_machine.vi"("State(s) in (\"\")"=w255) -> ("States Out"=w254:string)  [unwired: 14 in]
          }
          frame "UI: Cursor Set" {
            # "Argument"
            # "Initialize the User Interface, here.\n(this is called automatically, by the Macro: Init)"
            n88 = disable-structure shown="Default" {
              disable-tunnel: w258 -> [w263 w266]
              disable-tunnel: [w263 w265] -> w257
              disable-tunnel: w256 -> [_ w264]
              frame condition #0 {
              }
              frame condition #1 (active) {
                n89 = case shown="\"Busy\"" w264 {
                  tunnel: w266 -> [w268 w270]
                  tunnel: [w267 w269] -> w265
                  frame "Idle", Default {
                    n90 = call <vilib>:"Unset Busy.vi"("error in (no error)"=w268) -> ("error out"=w267:errorcluster)  [unwired: 10 in]
                  }
                  frame "Busy" {
                    n91 = call <vilib>:"Set Busy.vi"("error in (no error)"=w270) -> ("error out"=w269:errorcluster)  [unwired: 9 in, 1 out]
                  }
                }
              }
            }
            n92 = call <vilib>:"Add State(s) to Queue__jki_lib_state_machine.vi"("State(s) in (\"\")"=w262) -> ("States Out"=w261:string)  [unwired: 14 in]
          }
          frame "UI: Front Panel State" {
            # "Argument"
            # "Set Front Panel Open or Closed\n(Usage: \"UI: Front Panel State >> Open|Close\")"
            n93 = Unbundle By Name(w274) -> ("Core.Current VI Reference"=w273:refnum<vi>)
            n94 = disable-structure shown="Default" {
              disable-tunnel: w276 -> [w282 w305]
              disable-tunnel: [w281 w305] -> w275
              disable-tunnel: w273 -> [w280 _]
              disable-tunnel: w272 -> [w279 _]
              frame condition #0 (active) {
                n95 = case shown="\"Close\"" w279 {
                  tunnel: w282 -> [w286 w299]
                  tunnel: [w288 w300] -> w281
                  tunnel: w280 -> [w287 w297]
                  frame "Open", Default {
                    n96 = property class="VI"(reference=w287, error in=w286) -> (reference out=w284:refnum<vi>, error out=w285:errorcluster, "FP.State"=w283:T4)
                    n97 = case shown="\"Closed\"" w283 {
                      tunnel: [w291 w294] -> w288
                      tunnel: w285 -> [w290 w294]
                      tunnel: w284 -> [w289 _]
                      frame "Closed" {
                        n98 = invoke class="VI" method="FP.Open"(reference=w289, error in=w290, "Activate"=TRUE, "State"=T4."Standard") -> (error out=w291:errorcluster)  [unwired: 1 in, 4 out]
                      }
                      frame Default {
                      }
                    }
                  }
                  frame "Close" {
                    n99 = property class="VI"(reference=w297, error in=w299) -> (reference out=w296:refnum<vi>, error out=w298:errorcluster, "FP.State"=w295:T4)
                    n100 = case shown="Default" w295 {
                      tunnel: [w301 w304] -> w300
                      tunnel: w298 -> [w301 w303]
                      tunnel: w296 -> [_ w302]
                      frame "Invalid", "Closed" {
                      }
                      frame Default {
                        n101 = invoke class="VI" method="FP.Close"(reference=w302, error in=w303) -> (error out=w304:errorcluster)  [unwired: 1 in, 2 out]
                      }
                    }
                  }
                }
              }
              frame condition #1 {
              }
            }
            n102 = call <vilib>:"Add State(s) to Queue__jki_lib_state_machine.vi"("State(s) in (\"\")"=w278) -> ("States Out"=w277:string)  [unwired: 14 in]
          }
          frame "---------- Macro ----------" {
            # "Do not put any code in this frame.\n(It is a separator no-op. You can make a copy of this frame to create a new Macro frame)"
            n103 = call <vilib>:"Add State(s) to Queue__jki_lib_state_machine.vi"("State(s) in (\"\")"=w310) -> ("States Out"=w309:string)  [unwired: 14 in]
          }
          frame "Macro: Initialize" {
            w313 = "UI: Initialize\nMacro: Read UI Config\nAction: Open\n//UI: Front Panel State >> Open"  # UI: Initialize Macro: Read UI Config Action: Open //UI: Front Panel State >> Open
            # "Initialization Macro\n(This is called once, when the VI starts)"
            n104 = call <vilib>:"Add State(s) to Queue__jki_lib_state_machine.vi"("State(s) in Front (\"\")"="Data: Initialize\nInitialize Core Data\nEvents: Register", "State(s) in (\"\")"="Process: Sync", "State(s) at Back (\"\")"=w313) -> ("States Out"=w312:string)  [unwired: 12 in]
            n105 = call <vilib>:"Add State(s) to Queue__jki_lib_state_machine.vi"("State(s) in Front (\"\")"=w312, "State(s) in (\"\")"=w319) -> ("States Out"=w318:string)  [unwired: 13 in]
          }
          frame "Macro: Post Error Handling" {
            # "Clear Last Error?"
            n106 = Unbundle By Name(w321) -> ("Core.Last Error.remaining states"=w323:string, "Core.Shutdown?"=w324:bool)
            n107 = Unbundle By Name(w321) -> ("Core.Last Error.error"=w327:errorcluster)
            n108 = case shown="False" FALSE {
              tunnel: w327 -> [w335 _]
              tunnel: [w335 _] -> w326
              frame False {
              }
              frame True {
              }
            }
            n109 = case shown="False" w324 {
              tunnel: w323 -> [w332 w334]
              tunnel: [w332 w333] -> w320
              frame False {
                # "These are the remaining states (at the moment the error occured). States can be altered according to business logic."
                # "NOT SHUTTING DOWN"
              }
              frame True {
                # "Developer can decide to alter the states but should be aware that during the shutdown process, there are certain states that must be run for the SMO to properly shut itself (and this process) down. As such, one can add states to perform additional clean-ups, but should append the remaining state to be executed."
                # "SHUTTING DOWN"
                n110 = call <vilib>:"Add State(s) to Queue__jki_lib_state_machine.vi"("State(s) in (\"\")"=w334) -> ("States Out"=w333:string)  [unwired: 14 in]
              }
            }
            n111 = Bundle By Name(cluster=w321, "Core.Last Error.error"=w326) -> (w322:T10)
            n112 = call <vilib>:"Add State(s) to Queue__jki_lib_state_machine.vi"("State(s) in Front (\"\")"=w320, "State(s) in (\"\")"=w331) -> ("States Out"=w330:string)  [unwired: 13 in]
          }
          frame "Macro: Read UI Config" {
            # "Do not put any code in this frame.\n(It is a separator no-op. You can make a copy of this frame to create a new Macro frame)"
            n113 = call <vilib>:"Add State(s) to Queue__jki_lib_state_machine.vi"("State(s) in Front (\"\")"="Configuration: Initialize\nConfiguration: Read UI Config File\nUI: Update FP Controls" ("State(s) in Front (\"\")"), "State(s) in (\"\")"=w341) -> ("States Out"=w340:string)  [unwired: 13 in]
          }
          frame "Macro: Write UI Config" {
            # "Do not put any code in this frame.\n(It is a separator no-op. You can make a copy of this frame to create a new Macro frame)"
            n114 = call <vilib>:"Add State(s) to Queue__jki_lib_state_machine.vi"("State(s) in Front (\"\")"="Data: Set UI Cluster\nConfiguration: Write UI Config File" ("State(s) in Front (\"\")"), "State(s) in (\"\")"=w347) -> ("States Out"=w346:string)  [unwired: 13 in]
          }
          frame "Macro: Exit" {
            # "Exit Macro\n(This is called once, when the VI exits)"
            n115 = Unbundle By Name(w349) -> ("Core.Close Panel on Exit?"=w359:bool)
            n116 = Select(t="UI: Front Panel State >> Close", s=w359, f="" ("Empty String Constant")) -> (s? t:f=w356:string)
            n117 = call <vilib>:"Add State(s) to Queue__jki_lib_state_machine.vi"("State(s) in Front (\"\")"="Data: Cleanup\nEvents: Unregister\nProcess: Self Terminate", "State(s) in (\"\")"="Process: Sync", "State(s) at Back (\"\")"="Exit") -> ("States Out"=w351:string)  [unwired: 12 in]
            n118 = call <vilib>:"Add State(s) to Queue__jki_lib_state_machine.vi"("State(s) in Front (\"\")"="Action: Close\nMacro: Write UI Config", "State(s) in (\"\")"=w356, "State(s) at Back (\"\")"=w351) -> ("States Out"=w355:string)  [unwired: 12 in]
            n119 = call <vilib>:"Add State(s) to Queue__jki_lib_state_machine.vi"("State(s) in Front (\"\")"=w355, "State(s) in (\"\")"=w362) -> ("States Out"=w361:string)  [unwired: 13 in]
          }
          frame "---------- Process ----------" {
            # "Template Separator\n(You can make a copy of, or modify, this frame)"
            n120 = call <vilib>:"Add State(s) to Queue__jki_lib_state_machine.vi"("State(s) in (\"\")"=w367) -> ("States Out"=w366:string)  [unwired: 14 in]
          }
          frame "Process: Sync" {
            n121 = Unbundle By Name(w375) -> ("Instrument UI"=w371:refnum<class "Inst UI.RP100.lvclass">)
            n122 = call <vilib>:"WaitOnProcessSync.vi"("error in (no error)"=w370, "SMO"=w371) -> ("error out"=w369:errorcluster, "Don't run?"=w374:bool)  [unwired: 7 in, 1 out]
            n123 = Select(t="Data: Cleanup\nEvents: Unregister\nExit", s=w374, f="" ("Empty String Constant")) -> (s? t:f=w368:string)
            n124 = call <vilib>:"Add State(s) to Queue__jki_lib_state_machine.vi"("State(s) in Front (\"\")"=w368, "State(s) in (\"\")"=w378) -> ("States Out"=w377:string)  [unwired: 13 in]
          }
          frame "Process: Self Terminate" {
            n125 = Unbundle By Name(w380) -> ("Instrument UI"=w379:refnum<class "Inst UI.RP100.lvclass">)
            n126 = call <vilib>:"SelfTerminate.vi"("error in (no error)"=w382, "SMO in"=w379) -> ("error out"=w381:errorcluster)  [unwired: 8 in, 1 out]
            n127 = call <vilib>:"Add State(s) to Queue__jki_lib_state_machine.vi"("State(s) in (\"\")"=w385) -> ("States Out"=w384:string)  [unwired: 14 in]
          }
          frame "---------- Events ----------" {
            # "Template Separator\n(You can make a copy of, or modify, this frame)"
            n128 = call <vilib>:"Add State(s) to Queue__jki_lib_state_machine.vi"("State(s) in (\"\")"=w390) -> ("States Out"=w389:string)  [unwired: 14 in]
          }
          frame "Events: Register" {
            # "Expand to add\nmore events"
            # "Base Class Protected Events"
            n129 = Unbundle By Name(w407) -> ("Instrument UI"=w400:refnum<class "Inst UI.RP100.lvclass">, "Instrument"=w399:refnum<class "Inst.RP100.lvclass">)
            n130 = call <vilib>:"GetProtectedEvents.vi"("SMO"=w400) -> ("error out"=w403:errorcluster, "SMO Protected Events"=w405:T13)  [unwired: 8 in, 1 out]
            n131 = call <userlib>:"Instrument.GetPublicEvents.vi"("Instrument"=w399) -> ("error out"=w401:errorcluster, "Instrument Public Events"=w402:T14, "Instrument out"=w397:refnum<class "Inst.RP100.lvclass">)  [unwired: 8 in]
            n132 = call "Inst.RP100.GetPublicEvents.vi"("Inst.RP100 in"=w397) -> ("error out"=w396:errorcluster, "Inst.RP100 Public Events"=w398:T15, "Inst.RP100 out"=w393:refnum<class "Inst.RP100.lvclass">)  [unwired: 8 in]
            n133 = call <vilib>:"GetPublicEvents.vi"("SMO"=w393) -> ("error out"=w391:errorcluster, "Public Events"=w392:T16)  [unwired: 8 in, 1 out]
            n134 = register-events(w405, w402, w398, w392) -> (reference out=w406:refnum<event-registration>, error out=w395:errorcluster)  [unwired: 2 in]
            n135 = Merge Errors(w395, w391, w396, w401, w403, w394) -> (w404:errorcluster)
            n136 = call <vilib>:"Add State(s) to Queue__jki_lib_state_machine.vi"("State(s) in (\"\")"=w409) -> ("States Out"=w408:string)  [unwired: 14 in]
          }
          frame "Events: Unregister" {
            n137 = Unregister For Events(event registration refnum=w412, error in=w411) -> (error out=w410:errorcluster)
            n138 = call <vilib>:"Add State(s) to Queue__jki_lib_state_machine.vi"("State(s) in (\"\")"=w415) -> ("States Out"=w414:string)  [unwired: 14 in]
          }
          frame "---------- Configuration ----------" {
            # "Do not put any code in this frame.\n(It is a separator no-op. You can make a copy of this frame to create a new UI frame)"
            n139 = call <vilib>:"Add State(s) to Queue__jki_lib_state_machine.vi"("State(s) in (\"\")"=w420) -> ("States Out"=w419:string)  [unwired: 14 in]
          }
          frame "Configuration: Initialize" {
            # "Do not put any code in this frame.\n(It is a separator no-op. You can make a copy of this frame to create a new UI frame)"
            n140 = Unbundle By Name(w428) -> ("Configuration"=w426:refnum<class "Configuration.lvclass">, "Instrument"=w427:refnum<class "Inst.RP100.lvclass">)
            n141 = call <vilib>:"GetName.vi"("error in (no error)"=w430, "SMO"=w427) -> ("error out"=w429:errorcluster, "Name"=w431:string)  [unwired: 6 in, 2 out]
            n142 = call <userlib>:"Default Path.vi"("error in (no error)"=w429, "Folder Name [Application Name]"=w431, "Configuration in"=w426) -> ("error out"=w422:errorcluster, "Configuration out"=w425:refnum<class "Configuration.lvclass">)  [unwired: 7 in]
            n143 = call <userlib>:"Write Section.vi"("error in (no error)"=w422, "Section"="UI", "Configuration in"=w425) -> ("error out"=w421:errorcluster, "Configuration out"=w424:refnum<class "Configuration.lvclass">)  [unwired: 7 in]
            n144 = Bundle By Name(cluster=w428, "Configuration"=w424) -> (w432:T10)
            n145 = call <vilib>:"Add State(s) to Queue__jki_lib_state_machine.vi"("State(s) in (\"\")"=w435) -> ("States Out"=w434:string)  [unwired: 14 in]
          }
          frame "Configuration: Write UI Config File" {
            # "Do not put any code in this frame.\n(It is a separator no-op. You can make a copy of this frame to create a new Data frame)"
            n146 = Unbundle By Name(w440) -> ("Configuration"=w437:refnum<class "Configuration.lvclass">, "UI Cluster"=w439:T9)
            n147 = call <userlib>:"Write Configuration.vi"("error in (no error)"=w436, "Variant"=w439, "Configuration in"=w437) -> ("error out"=w438:errorcluster)  [unwired: 7 in, 1 out]
            n148 = call <vilib>:"Add State(s) to Queue__jki_lib_state_machine.vi"("State(s) in (\"\")"=w443) -> ("States Out"=w442:string)  [unwired: 14 in]
          }
          frame "Configuration: Read UI Config File" {
            # "Do not put any code in this frame.\n(It is a separator no-op. You can make a copy of this frame to create a new UI frame)"
            n149 = Unbundle By Name(w446) -> ("UI Cluster"=w449:T9, "Configuration"=w452:refnum<class "Configuration.lvclass">)
            n150 = call <userlib>:"Read Configuration.vi"("INI Fomatted Cluster Type"=w449, "error in (no error)"=w448, "Configuration in"=w452) -> ("error out"=w451:errorcluster, "Configuration"=w450:variant)  [unwired: 6 in, 1 out]
            n151 = Variant To Data(error in=w451, type=w449, Variant=w450) -> (data=w445:T9, error out=w447:errorcluster)
            n152 = Bundle By Name(cluster=w446, "UI Cluster"=w445) -> (w444:T10)
            n153 = call <vilib>:"Add State(s) to Queue__jki_lib_state_machine.vi"("State(s) in (\"\")"=w455) -> ("States Out"=w454:string)  [unwired: 14 in]
          }
          frame "---------- Action ----------" {
            n154 = Unbundle By Name(w457) -> ("Instrument"=w458:refnum<class "Inst.RP100.lvclass">)
            n155 = Bundle By Name(cluster=w457, "Instrument"=w458) -> (w456:T10)
            n156 = call <vilib>:"Add State(s) to Queue__jki_lib_state_machine.vi"("State(s) in (\"\")"=w462) -> ("States Out"=w461:string)  [unwired: 14 in]
          }
          frame "Action: Notify UI Closed" {
            # "Notify that the UI has been closed"
            n157 = Unbundle By Name(w463) -> ("Instrument UI"=w466:refnum<class "Inst UI.RP100.lvclass">)
            n158 = call <vilib>:"Hide.vi"("error in (no error)"=w465, "SMO.UI"=w466) -> ("error out"=w464:errorcluster)  [unwired: 8 in, 1 out]
            n159 = call <vilib>:"Add State(s) to Queue__jki_lib_state_machine.vi"("State(s) in (\"\")"=w469) -> ("States Out"=w468:string)  [unwired: 14 in]
          }
          frame "Action: getAll" {
            n160 = Unbundle By Name(w473) -> ("getAll"=w471:T8, "Instrument"=w476:refnum<class "Inst.RP100.lvclass">)
            n161 = call "GET ALL.vim"("type"=w471, "error in (no error)"=w474, "Instrument in"=w476) -> ("error out"=w478:errorcluster, "getAll"=w470:T8, "Instrument out"=w472:refnum<class "Inst.RP100.lvclass">)  [unwired: 6 in]
            n162 = Bundle By Name(cluster=w473, "Instrument"=w472, "getAll"=w470) -> (w475:T10)
            n163 = call <vilib>:"Add State(s) to Queue__jki_lib_state_machine.vi"("State(s) in Front (\"\")"="" ("State(s) in Front (\"\")"), "State(s) in (\"\")"=w481) -> ("States Out"=w480:string)  [unwired: 13 in]
          }
          frame "Action: Open" {
            n164 = Unbundle By Name(w488) -> ("Instrument"=w486:refnum<class "Inst.RP100.lvclass">)
            n165 = call <userlib>:"Write Client Type.vi"("error in (no error)"=w483, "Client Type"=Client_Type--Enum."Local", "Instrument in"=w486) -> ("error out"=w484:errorcluster, "Instrument out"=w485:refnum<class "Inst.RP100.lvclass">)  [unwired: 7 in]
            n166 = call-dynamic "Open.vi"("error in (no error)"=w484, "Inst.RP100 in"=w485) -> ("error out"=w491:errorcluster, "Inst.RP100 out"=w487:refnum<class "Inst.RP100.lvclass">)  [unwired: 8 in]
            n167 = Bundle By Name(cluster=w488, "Instrument"=w487) -> (w489:T10)
            n168 = call <vilib>:"Add State(s) to Queue__jki_lib_state_machine.vi"("State(s) in Front (\"\")"="" ("State(s) in Front (\"\")"), "State(s) in (\"\")"=w494) -> ("States Out"=w493:string)  [unwired: 13 in]
          }
          frame "Action: Close" {
            n169 = Unbundle By Name(w496) -> ("Instrument"=w499:refnum<class "Inst.RP100.lvclass">)
            n170 = call-dynamic "Close.vi"("error in (no error)"=w497, "Inst.RP100 in"=w499) -> ("error out"=w501:errorcluster, "Inst.RP100 out"=w495:refnum<class "Inst.RP100.lvclass">)  [unwired: 8 in]
            n171 = Bundle By Name(cluster=w496, "Instrument"=w495) -> (w498:T10)
            n172 = call <vilib>:"Add State(s) to Queue__jki_lib_state_machine.vi"("State(s) in Front (\"\")"="" ("State(s) in Front (\"\")"), "State(s) in (\"\")"=w504) -> ("States Out"=w503:string)  [unwired: 13 in]
          }
          frame "Action: Send Message to Instrument" {
            # "Send a message (command, data, etc) to the Instrument:process.vi"
            n173 = Unbundle By Name(w509) -> ("Instrument"=w508:refnum<class "Inst.RP100.lvclass">)  [unwired: 1 out]
            n174 = call <userlib>:"Instrument.MessageToProcess.vi"("error in (no error)"=w506, "Instrument"=w508) -> ("error out"=w505:errorcluster, "Instrument out"=w507:refnum<class "Inst.RP100.lvclass">)  [unwired: 8 in]
            n175 = Bundle By Name(cluster=w509, "Instrument"=w507) -> (w510:T10)
            n176 = call <vilib>:"Add State(s) to Queue__jki_lib_state_machine.vi"("State(s) in Front (\"\")"="" ("State(s) in Front (\"\")"), "State(s) in (\"\")"=w514) -> ("States Out"=w513:string)  [unwired: 13 in]
          }
          frame "Action: Send Message to Child" {
            # "Send a message (command, data, etc) to the Instrument.Child:process.vi"
            n177 = Unbundle By Name(w519) -> ("Instrument"=w518:refnum<class "Inst.RP100.lvclass">)  [unwired: 1 out]
            n178 = call "Inst.RP100.MessageToProcess.vi"("error in (no error)"=w516, "Inst.RP100 in"=w518) -> ("error out"=w515:errorcluster, "Inst.RP100 out"=w517:refnum<class "Inst.RP100.lvclass">)  [unwired: 8 in]
            n179 = Bundle By Name(cluster=w519, "Instrument"=w517) -> (w520:T10)
            n180 = call <vilib>:"Add State(s) to Queue__jki_lib_state_machine.vi"("State(s) in Front (\"\")"="" ("State(s) in Front (\"\")"), "State(s) in (\"\")"=w524) -> ("States Out"=w523:string)  [unwired: 13 in]
          }
        }
      }
    }
    frame Error {
    }
  }
  n181 = call-parent "Process.vi"("error in"=w5, "Instrument UI in"=w4) -> ("error out"=w2:errorcluster, "Instrument UI out"=→"Inst UI.RP100 out":refnum<class "Inst UI.RP100.lvclass">)  [unwired: 8 in]
  n182 = Merge Errors(w2, w1) -> (→"error out":errorcluster)
